vi "GlobalGetAOTFOnOff.vi"() -> ()   [LabVIEW 2011]
panel:
  out "GetAOTF":bool
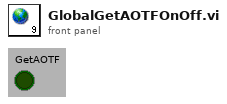
[diagram p1: front panel]
diagram:
